vi "OAT Tachless Band Limit of Chkpoints.vi"(9 "interested orders list":dbl[](array[numeric]) format="%.2f", 10 "Current Order":dbl format="%.2f", 11 "speed profile":T1 {"speed [RPM]" format="%.2f"; "time [s]" format="%.2f"}) -> (1 "interested orders":cluster{"X":dbl[], "Y":dbl[]}[](array[cluster]) {"Y" format="%.2f"; "X" format="%.2f"}, 2 "Lower Limit":cluster{"X":dbl[], "Y":dbl[]} {"Y" format="%.2f"; "X" format="%.2f"}, 3 "Upper Limit":cluster{"X":dbl[], "Y":dbl[]} {"Y" format="%.2f"; "X" format="%.2f"})   [LabVIEW 2017, in "SoundVib_Tachless.lvlib"]
uses:
  <vilib>/addons/Sound and Vibration/Order Analysis/Tachless/SoundVib_Tachless.lvlib
  <vilib>/addons/Sound and Vibration/Order Analysis/Tach Process/SubVIs/speed profile.ctl
  <vilib>/addons/Sound and Vibration/Order Analysis/Tach Process/SoundVib_TachProcess.lvlib
panel:
  in  "unit":u16
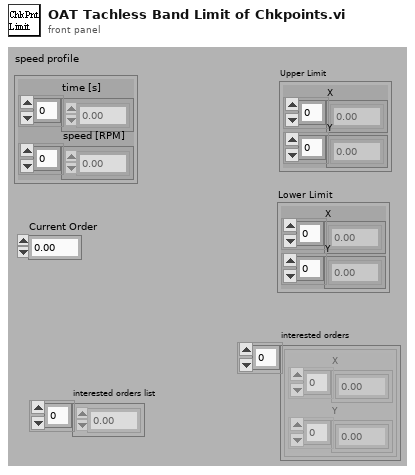
[diagram p1: front panel]
types:
  T1 = typedef "SoundVib_TachProcess.lvlib/speed profile.ctl" = cluster{"time [s]":dbl[], "speed [RPM]":dbl[]}
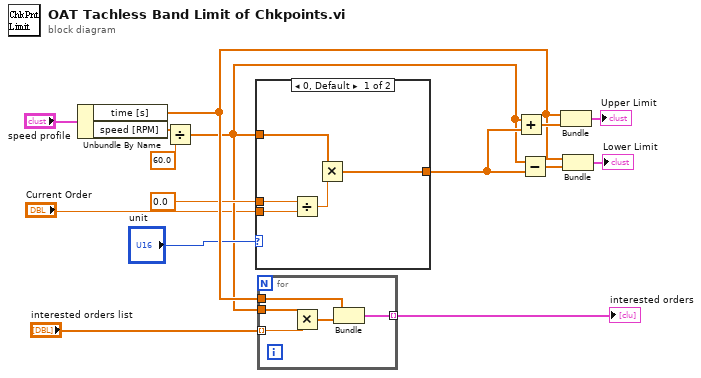
[diagram p0: block diagram]
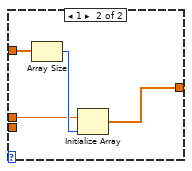
[diagram p2: hidden frame]
diagram:
  n1 = Unbundle By Name("speed profile") -> ("time [s]"=w8:dbl[], "speed [RPM]"=w12:dbl[])
  n2 = Divide(x=w12, y=60.0) -> (x/y=w3:dbl[])
  n3 = case shown="0, Default" "unit" {
    tunnel: [w16 w21] -> w11
    tunnel: 0.0 ("Bandwidth") -> [w20 w22]
    tunnel: w3 -> [w18 w24]
    tunnel: "Current Order" -> [w19 _]
    frame 0, Default {
      n4 = Divide(x=w20, y=w19) -> (x/y=w17:dbl)
      n5 = Multiply(x=w18, y=w17) -> (x*y=w16:dbl[])
    }
    frame 1 {
      n6 = Array Size(array=w24) -> (size(s)=w23:i32)
      n7 = Initialize Array(w22, w23) -> (w21:dbl[])
    }
  }
  n8 = for {
    tunnel: "interested orders list" -> [w29] mode=indexing
    tunnel: w3 -> [w25]
    tunnel: w8 -> [w28]
    tunnel: [w27] -> w13 mode=indexing
    n9 = Multiply(x=w25, y=w29) -> (x*y=w26:dbl[])
    n10 = Bundle("time [s]"=w28, w26) -> (w27:cluster{"time [s]":dbl[], dbl[]})  [unwired: 1 in]
  }
  "interested orders" <- w13
  n11 = Add(x=w3, y=w11) -> (x+y=w9:dbl[])
  n12 = Subtract(x=w3, y=w11) -> (x-y=w10:dbl[])
  n13 = Bundle("time [s]"=w8, w9) -> (→"Upper Limit":cluster{"time [s]":dbl[], dbl[]})  [unwired: 1 in]
  n14 = Bundle("time [s]"=w8, w10) -> (→"Lower Limit":cluster{"time [s]":dbl[], dbl[]})  [unwired: 1 in]
